vi "Write AIP Status.vi"(8 "error in (no error)":errorcluster, 10 "AIP Status":T1, 11 "RDS State in":refnum<class "RDS State.lvclass">) -> (0 "error out":errorcluster, 3 "RDS State out":refnum<class "RDS State.lvclass">)   [LabVIEW 2015, in "RDS Child Messages.lvlib" / "RDS State.lvclass"]
uses:
  RDS State.lvclass
  Libraries/RDS Instruments/AIP/AIP Status.ctl
  Libraries/RDS Instruments/AIP/AIP States.ctl
  RDS State.lvclass/RDS State.ctl
  Libraries/RDS Instruments/RDS Instrument Library.lvlib
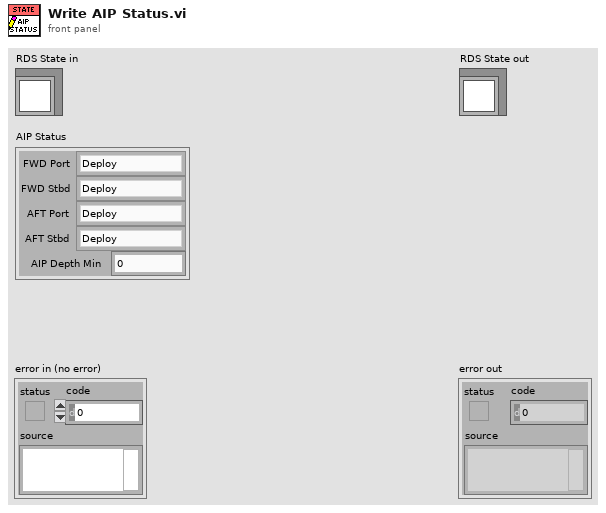
[diagram p1: front panel]
types:
  T1 = typedef "RDS Instrument Library.lvlib/AIP Status.ctl" = cluster{"FWD Port":T2, "FWD Stbd":T2, "AFT Port":T2, "AFT Stbd":T2, "AIP Depth Min":u8}
  T2 = typedef "RDS Instrument Library.lvlib/AIP States.ctl" = enum16{"Deploy", "Deploying", "Deployed", "Stow", "Stowing", "Stowed", "Fault", "brakeOnStow", "breakOnDeploy", "Stopped", "Stopping"}
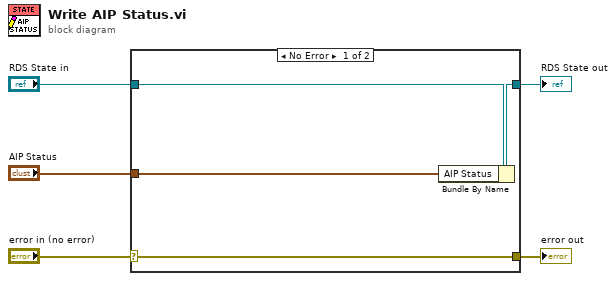
[diagram p0: block diagram]
diagram:
  n1 = case shown="No Error" "error in (no error)" {
    selector: "error in (no error)" -> [w9 w10]
    tunnel: [w9 w10] -> w4
    tunnel: [w7 w11] -> w2
    tunnel: "RDS State in" -> [w8 w11]
    tunnel: "AIP Status" -> [w6 _]
    frame No Error {
      n2 = Bundle By Name(cluster=w8, "AIP Status"=w6) -> (w7:refnum<class "RDS State.lvclass">)
    }
    frame Error {
    }
  }
  "error out" <- w4
  "RDS State out" <- w2
